vi "Write Core.vi"(8 "error in (no error)":errorcluster, 10 "PV":refnum<class "PV.lvclass">, 11 "PVConnection in":refnum<class "DSConnection.lvclass">) -> (0 "error out":errorcluster, 3 "PVConnection out":refnum<class "DSConnection.lvclass">)   [LabVIEW 2015, in "CS++ProcessVariables.lvlib" / "DSConnection.lvclass"]
doc: "Publish a process variable."
uses:
  DSConnection.lvclass
  ProcessVariable/PV.lvclass
  DSConnection.lvclass/DSConnection.ctl
  ProcessVariable/PV.lvclass/PV.ctl
  Libraries/Utilities/CS++Utilities.lvlib
  PVConnection/PVConnection.lvclass
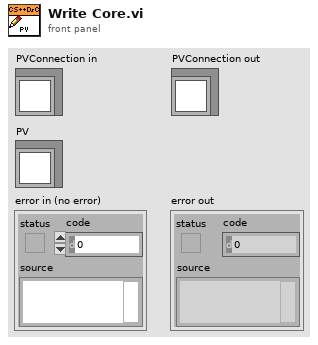
[diagram p1: front panel]
types:
  T1 = cluster{"Read Access":enum8{"Allowed", "Required", "None"}, "Write Access":enum8{"Allowed", "Required", "None"}}
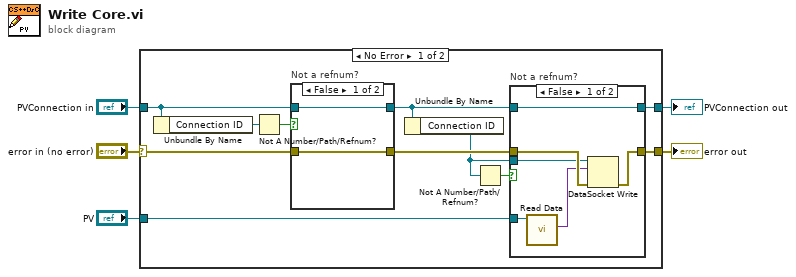
[diagram p0: block diagram]
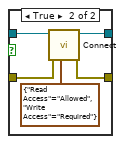
[diagram p2: hidden frame]
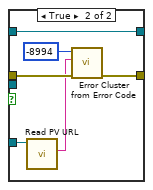
[diagram p3: hidden frame]
diagram:
  n1 = case shown="No Error" "error in (no error)" {
    selector: "error in (no error)" -> [w11 w37]
    tunnel: [w16 w37] -> w5
    tunnel: [w15 w36] -> w4
    tunnel: "PV" -> [w6 _]
    tunnel: "PVConnection in" -> [w10 w36]
    frame No Error {
      n2 = Unbundle By Name(w10) -> ("Connection ID"=w13:refnum<k13>)
      n3 = Not A Number/Path/Refnum?(number/path/refnum=w13) -> (NaN/Path/Refnum?=w14:bool)
      n4 = case "Not a refnum?" shown="False" w14 {
        tunnel: w10 -> [w17 w23]
        tunnel: [w17 w22] -> w9
        tunnel: w11 -> [w18 w21]
        tunnel: [w18 w20] -> w12
        frame False {
        }
        frame True {
          n5 = call "Connect.vi"("Access (R/W allowed)"=T1 {"Read Access"=enum."Allowed", "Write Access"=enum."Required"}, "Error In"=w21, "PVConnection in"=w23) -> ("Error Out"=w20:errorcluster, "PVConnection out"=w22:refnum<class "DSConnection.lvclass">)  [unwired: 7 in]
        }
      }
      n6 = Unbundle By Name(w9) -> ("Connection ID"=w7:refnum<k13>)
      n7 = Not A Number/Path/Refnum?(number/path/refnum=w7) -> (NaN/Path/Refnum?=w8:bool)
      n8 = case "Not a refnum?" shown="False" w8 {
        tunnel: [w27 w32] -> w16
        tunnel: [w29 w35] -> w15
        tunnel: w9 -> [w29 w35]
        tunnel: w12 -> [w28 w33]
        tunnel: w6 -> [w26 w31]
        tunnel: w7 -> [w24 _]
        frame False {
          n9 = call "Read Data.vi"("PV in"=w26) -> ("Data"=w25:variant)  [unwired: 8 in, 2 out]
          n10 = DataSocket Write(8:w28, 10:w25, 11:w24) -> (0:w27:errorcluster)  [unwired: 1 in, 2 out]
        }
        frame True {
          n11 = call "Read PV URL.vi"("PV in"=w31) -> ("PV URL"=w30:string)  [unwired: 8 in, 2 out]
          n12 = call "Error Cluster from Error Code.vi"("Error In"=w33, "Error Message (\"\")"=w30, "Error Code (0)"=-8994 ("error code (0)")) -> ("Error Out"=w32:errorcluster)  [unwired: 8 in]
        }
      }
    }
    frame Error {
    }
  }
  "error out" <- w5
  "PVConnection out" <- w4
